vi "fruit.caught.vi"(8 "error in (no error)":errorcluster, 11 "Game Board in":refnum<class "Game Board.lvclass">) -> (0 "error out":errorcluster, 2 "Fruit Caught":bool, 3 "Game Board out":refnum<class "Game Board.lvclass">)   [LabVIEW 2020, in "Game Board.lvclass"]
uses:
  Game Board.lvclass
  Game Board.lvclass/Game Board.ctl
  Snake/Snake.lvclass/Snake.ctl
  Fruit/Fruit.lvclass
  Snake/Snake.lvclass
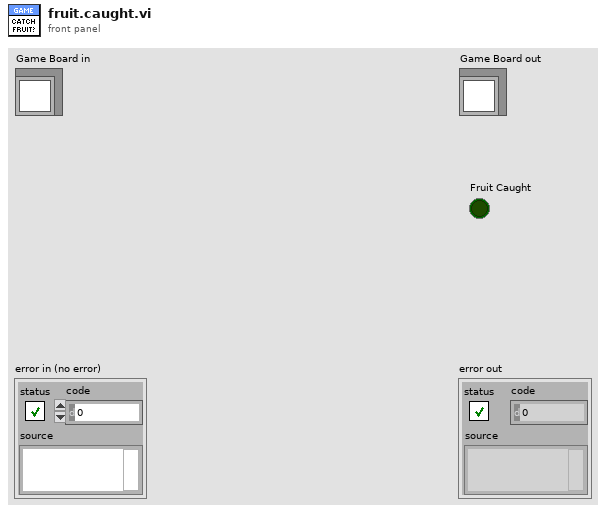
[diagram p1: front panel]
types:
  T1 = typedef "Coordinates.ctl" = cluster{"X":i32, "Y":i32}
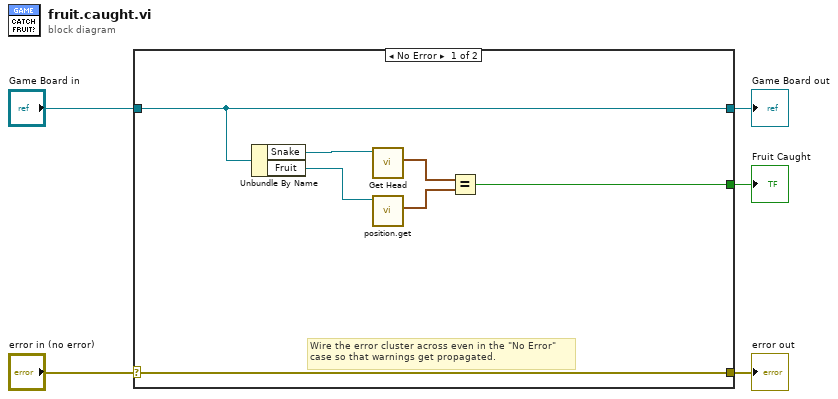
[diagram p0: block diagram]
diagram:
  n1 = case shown="No Error" "error in (no error)" {
    selector: "error in (no error)" -> [w12 w14]
    tunnel: [w12 w14] -> w4
    tunnel: [w6 w13] -> w2
    tunnel: "Game Board in" -> [w6 w13]
    tunnel: [w7 _] -> w1
    frame No Error {
      # "Wire the error cluster across even in the \"No Error\"\ncase so that warnings get propagated."
      n2 = Unbundle By Name(w6) -> ("Snake"=w11:refnum<class "Snake.lvclass">, "Fruit"=w10:refnum<class "Fruit.lvclass">)
      n3 = call "Get Head.vi"("Snake in"=w11) -> ("Coordinates"=w9:T1)  [unwired: 10 in]
      n4 = call-dynamic "position.get.vi"("Fruit in"=w10) -> ("Coordinates"=w8:T1)  [unwired: 10 in]
      n5 = Equal?(x=w9, y=w8) -> (x = y?=w7:bool)
    }
    frame Error {
    }
  }
  "error out" <- w4
  "Game Board out" <- w2
  "Fruit Caught" <- w1
